vi "Send Set Grid Value Using Coordinates.vi"(6 "Cell Value":bool, 7 "Message Priority (Normal)":T1=enum."Normal", 8 "error in (no error)":errorcluster, 9 "Row":u32, 10 "Column":u32, 11 "Message Enqueuer":refnum<class "Message Enqueuer.lvclass">) -> (0 "error out":errorcluster, 3 "Message Enqueuer out":refnum<class "Message Enqueuer.lvclass">)   [LabVIEW 2024, in "Grid Screen.lvlib" / "Set Grid Value Using Coordinates Msg.lvclass"]
doc: "This VI sends the message to an actor."
uses:
  Set Grid Value Using Coordinates Msg.lvclass
  <vilib>/ActorFramework/Message Enqueuer/Message Enqueuer.lvclass
  <vilib>/ActorFramework/Message Enqueuer/Message Priority.ctl
  C:/Program Files/National Instruments/LabVIEW 2024/vi.lib/ActorFramework/Message/Message.lvclass
  Set Grid Value Using Coordinates Msg.lvclass/Set Grid Value Using Coordinates Msg.ctl
  <vilib>/ActorFramework/Message Enqueuer/Message Enqueuer.lvclass/Message Enqueuer.ctl
  <vilib>/ActorFramework/Message Priority Queue/Priority Enqueue.vi
  C:/Users/ekerry/Documents/challenge-of-champions/MC Screen/Grid Screen Messages/Set Grid Value Using Coordinates Msg/Set Grid Value Using Coordinates Msg.lvclass
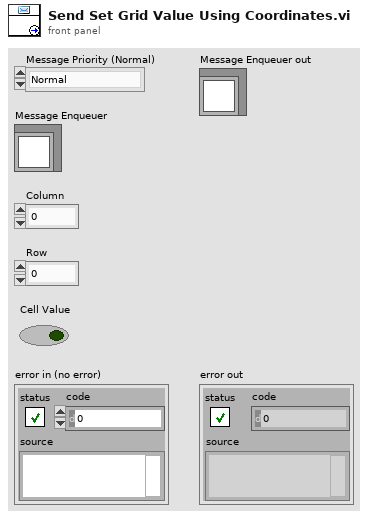
[diagram p1: front panel]
types:
  T1 = typedef "Actor Framework.lvlib/Message Enqueuer.lvclass/Message Priority.ctl" = enum16{"Low", "Normal", "High"}
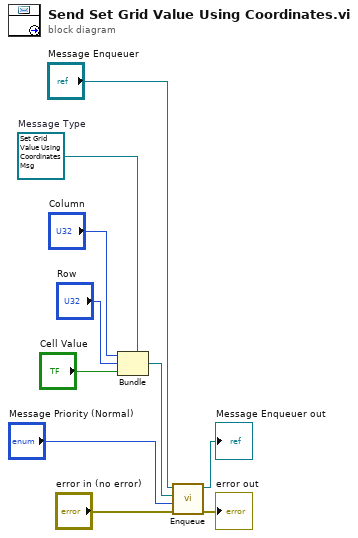
[diagram p0: block diagram]
diagram:
  w7 = refnum<class "Set Grid Value Using Coordinates Msg.lvclass"> refnum  # Message Type
  n1 = Bundle(cluster=w7, "Column", "Row", "Cell Value") -> (w6:refnum<class "Set Grid Value Using Coordinates Msg.lvclass">)
  n2 = call <vilib>:"Enqueue.vi"("error in (no error)"="error in (no error)", "Message Priority (Normal)"="Message Priority (Normal)", "Message"=w6, "Message Enqueuer in"="Message Enqueuer") -> ("error out"=→"error out":errorcluster, "Message Enqueuer in"=→"Message Enqueuer out":refnum<class "Message Enqueuer.lvclass">)  [unwired: 6 in]
